vi "convFromConfigData.vi"(5 "Config in":T1) -> (2 "Config out":u8[](array[numeric]))   [LabVIEW 2015, in "TPVG_DLL.lvlib"]
doc: "------------------------------------------\nAuthor: Dang Lam\nEmail: danglamtd@gmail.com"
uses:
  TPVG_DLL.lvlib
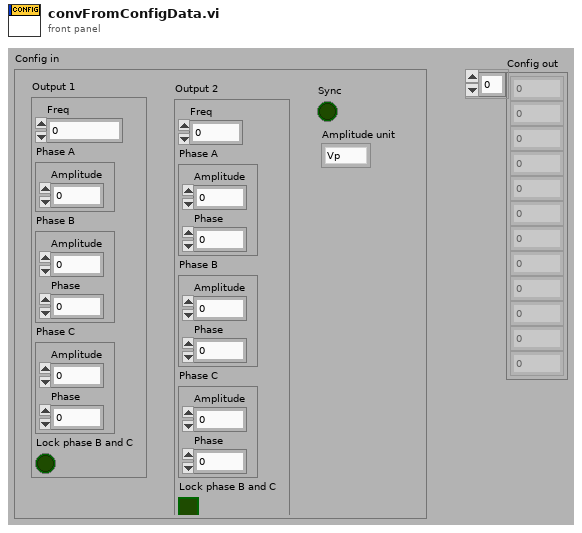
[diagram p1: front panel]
types:
  T1 = cluster{"Output 1":cluster{"Freq":sgl, "Phase A":cluster{"Amplitude":sgl}, "Phase B":cluster{"Amplitude":sgl, "Phase":sgl}, "Phase C":cluster{"Amplitude":sgl, "Phase":sgl}, "Lock":bool}, "Output 2":cluster{"Freq":sgl, "Phase A":cluster{"Amplitude":sgl, "Phase":sgl}, "Phase B":cluster{"Amplitude":sgl, "Phase":sgl}, "Phase C":cluster{"Amplitude":sgl, "Phase":sgl}, "Lock":bool}, "Sync":bool, "Amplitude unit":enum16{"Vp", "Vp-p", "Vrms"}}
  T2 = cluster{"Freq":sgl, "Phase A":cluster{"Amplitude":sgl}, "Phase B":cluster{"Amplitude":sgl, "Phase":sgl}, "Phase C":cluster{"Amplitude":sgl, "Phase":sgl}, "Lock":bool}
  T3 = cluster{"Freq":sgl, "Phase A":cluster{"Amplitude":sgl, "Phase":sgl}, "Phase B":cluster{"Amplitude":sgl, "Phase":sgl}, "Phase C":cluster{"Amplitude":sgl, "Phase":sgl}, "Lock":bool}
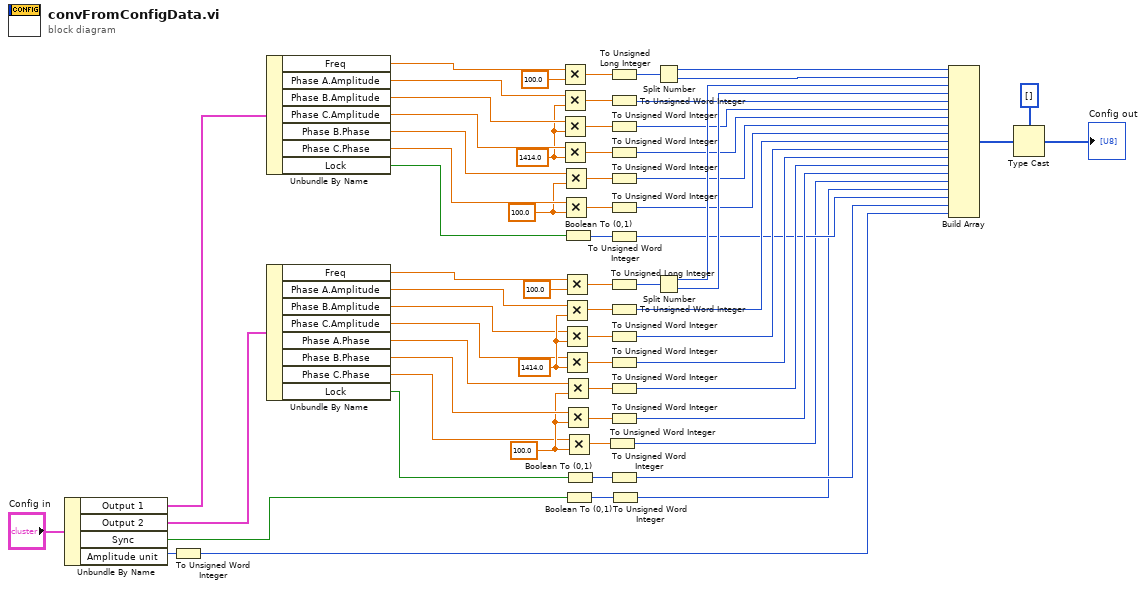
[diagram p0: block diagram]
diagram:
  w7 = sgl 100.0 ("y")
  w53 = sgl 1414.0 ("y")
  w55 = sgl 100.0 ("y")
  w58 = sgl 1414.0 ("y")
  n1 = Unbundle By Name("Config in") -> ("Output 1"=w65:T2, "Output 2"=w64:T3, "Sync"=w31:bool, "Amplitude unit"=w2:enum16{"Vp", "Vp-p", "Vrms"})
  n2 = To Unsigned Word Integer(number=w2) -> (unsigned 16bit integer=w1:u16)
  n3 = Unbundle By Name(w65) -> ("Freq"=w63:sgl, "Phase A.Amplitude"=w61:sgl, "Phase B.Amplitude"=w60:sgl, "Phase C.Amplitude"=w59:sgl, "Phase B.Phase"=w57:sgl, "Phase C.Phase"=w56:sgl, "Lock"=w54:bool)
  n4 = Unbundle By Name(w64) -> ("Freq"=w51:sgl, "Phase A.Amplitude"=w50:sgl, "Phase B.Amplitude"=w49:sgl, "Phase C.Amplitude"=w48:sgl, "Phase A.Phase"=w47:sgl, "Phase B.Phase"=w8:sgl, "Phase C.Phase"=w6:sgl, "Lock"=w46:bool)
  n5 = Multiply(x=w63, y=sgl 100.0) -> (x*y=w45:sgl)
  n6 = Multiply(x=w61, y=w58) -> (x*y=w40:sgl)
  n7 = Multiply(x=w60, y=w58) -> (x*y=w39:sgl)
  n8 = Multiply(x=w59, y=w58) -> (x*y=w38:sgl)
  n9 = Multiply(x=w57, y=w55) -> (x*y=w43:sgl)
  n10 = Multiply(x=w56, y=w55) -> (x*y=w42:sgl)
  n11 = Multiply(x=w51, y=sgl 100.0) -> (x*y=w44:sgl)
  n12 = Multiply(x=w50, y=w53) -> (x*y=w36:sgl)
  n13 = Multiply(x=w49, y=w53) -> (x*y=w35:sgl)
  n14 = Multiply(x=w48, y=w53) -> (x*y=w34:sgl)
  n15 = Boolean To (0,1)(Boolean=w54) -> (0, 1=w37:i16)
  n16 = Multiply(x=w47, y=w7) -> (x*y=w33:sgl)
  n17 = Multiply(x=w8, y=w7) -> (x*y=w32:sgl)
  n18 = Multiply(x=w6, y=w7) -> (x*y=w5:sgl)
  n19 = Boolean To (0,1)(Boolean=w31) -> (0, 1=w30:i16)
  n20 = Boolean To (0,1)(Boolean=w46) -> (0, 1=w41:i16)
  n21 = To Unsigned Word Integer(number=w5) -> (unsigned 16bit integer=w4:u16)
  n22 = To Unsigned Long Integer(number=w45) -> (unsigned 32bit integer=w29:u32)
  n23 = To Unsigned Word Integer(number=w40) -> (unsigned 16bit integer=w23:u16)
  n24 = To Unsigned Word Integer(number=w39) -> (unsigned 16bit integer=w22:u16)
  n25 = To Unsigned Word Integer(number=w38) -> (unsigned 16bit integer=w21:u16)
  n26 = To Unsigned Word Integer(number=w43) -> (unsigned 16bit integer=w20:u16)
  n27 = To Unsigned Word Integer(number=w42) -> (unsigned 16bit integer=w19:u16)
  n28 = To Unsigned Word Integer(number=w37) -> (unsigned 16bit integer=w13:u16)
  n29 = To Unsigned Long Integer(number=w44) -> (unsigned 32bit integer=w28:u32)
  n30 = To Unsigned Word Integer(number=w36) -> (unsigned 16bit integer=w18:u16)
  n31 = To Unsigned Word Integer(number=w35) -> (unsigned 16bit integer=w17:u16)
  n32 = To Unsigned Word Integer(number=w34) -> (unsigned 16bit integer=w16:u16)
  n33 = To Unsigned Word Integer(number=w33) -> (unsigned 16bit integer=w15:u16)
  n34 = To Unsigned Word Integer(number=w32) -> (unsigned 16bit integer=w14:u16)
  n35 = To Unsigned Word Integer(number=w41) -> (unsigned 16bit integer=w12:u16)
  n36 = To Unsigned Word Integer(number=w30) -> (unsigned 16bit integer=w3:u16)
  n37 = Split Number(x=w29) -> (hi(x)=w27:u16, lo(x)=w26:u16)
  n38 = Split Number(x=w28) -> (hi(x)=w25:u16, lo(x)=w24:u16)
  n39 = Build Array(w27, w26, w25, w24, w23, w22, w21, w20, w19, w18, w17, w16, w15, w14, w4, w3, w13, w12, w1) -> (w11:u16[])
  n40 = Type Cast(type=u8[] [], x=w11) -> (*(type *) &x=→"Config out":u8[])
